vi "twoDtext2array_wPath(dbl).vi"(11 "String":string="\\voltsPerGram.txt") -> (3 "all rows":dbl[][](array[numeric]))   [LabVIEW 2017]
uses:
  <vilib>/Utility/file.llb/Read Delimited Spreadsheet (DBL).vi
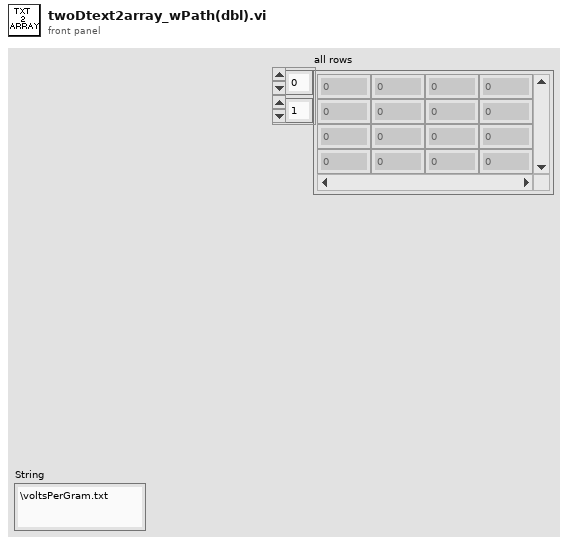
[diagram p1: front panel]
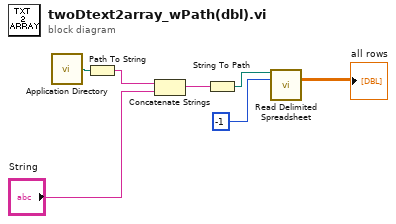
[diagram p0: block diagram]
diagram:
  n1 = call <vilib>:"Application Directory.vi"() -> ("Application Directory"=w6:path)
  n2 = Path To String(path=w6) -> (string=w5:string)
  n3 = Concatenate Strings(w5, "String") -> (w4:string)
  n4 = String To Path(string=w4) -> (path=w3:path)
  n5 = call-poly <vilib>:"Read Delimited Spreadsheet.vi"("file path (dialog if empty)"=w3, "number of rows (all:-1)"=-1) -> ("all rows"=→"all rows":dbl[][])  [unwired: 8 in, 5 out]
